vi "V2.4.vi"() -> ()   [LabVIEW 2023]
uses:
  c7928293-0f33-4b54-9085-86d351d5847f.vi
  e7d9e3fd-40eb-4ac7-a8e8-0c749fa94dbf.vi
  <vilib>/Utility/file.llb/Read Delimited Spreadsheet (DBL).vi
  <vilib>/Utility/file.llb/Read Delimited Spreadsheet (string).vi
  <vilib>/Analysis/4window.llb/Symmetric Window (DBL).vi
  <vilib>/Analysis/NI_AAL_SigProc.lvlib
  <vilib>/Analysis/NI_AALPro.lvlib
  <vilib>/Analysis/NI_AALBase.lvlib
panel:
  out "Pics + Index (nvl fct)":dbl[][](array[numeric])
  out "Vallées + Index (nvl fct)":dbl[][](array[numeric])
  out "Var V2V":dbl caption="variance" format="%0.2f"
  out "ET V2V":dbl caption="écart-type" format="%0.2f"
  out "Moy V2V":dbl caption="moyenne" format="%0.2f"
  out "V2V (nvl fct)":dbl[](array[numeric])
  out "Vallées + index DOUBLONS":dbl[][](array[numeric])
  out "var P2P":dbl caption="variance" format="%0.2f"
  out "ET P2P":dbl caption="écart-type" format="%0.2f"
  out "moy P2P":dbl caption="moyenne" format="%0.2f"
  out "P2P (nvl fct) 2":dbl[](array[numeric])
  out "Pics + index DOUBLONS":dbl[][](array[numeric])
  out "Graphe":dbl[](graph)
  out "pente":dbl[](graph)
  out "Pentes":dbl[](array[numeric]) format="%#.6g"
  out "Box moy de 20":dbl[](array[numeric])
  out "Pics Détectés 3":i32 caption="nb trouvé"
  out "Vallées Détectées 3":i32 caption="nb trouvé"
  out "Largeur V":dbl
  out "Seuil V":dbl
  out "Largeur P":dbl
  out "Seuil P":dbl
  out "variance V":dbl caption="variance" format="%0.2f"
  out "standard deviation V":dbl caption="écart-type" format="%0.2f"
  out "mean V":dbl caption="moyenne" format="%0.2f"
  out "Longueur V2V":i32[](array[numeric])
  out "variance P":dbl caption="variance" format="%0.2f"
  out "standard deviation P":dbl caption="écart-type" format="%0.2f"
  out "mean P":dbl caption="moyenne" format="%0.2f"
  out "Longueur P2P":i32[](array[numeric])
  out "Index Vallées":dbl[](array[numeric])
  out "Index Pics":dbl[](array[numeric])
  out "Longueurs SC 2 SC":i32[](graph)
  out "variance":dbl format="%0.2f"
  out "standard deviation 2":dbl caption="écart-type" format="%0.2f"
  out "mean 3":dbl caption="moyenne" format="%0.2f"
  out "First Val of traces":dbl[](array[numeric])
  out "Tableau":dbl[][](array[numeric])
  out "SC1 s":i32[](array[numeric])
  out "Nb de pas (g et dr)":i32
  out "Graphe de signaux mixte":dbl[][](graph)
  out "Cluster":cluster{"SC1":i32, "Aerial":i32, "SC 2":i32}
  out "Longueur de chaque pas (SC 2 SC)":i32[](array[numeric])
  out "Etapes des pas":cluster{"SC1":i32, "Aerial":i32, "SC 2":i32}[](array[cluster])
  out "All data SC/DC/Aerial":string[](array[string])
  out "W condi ?":bool
  out "V target":dbl
  out "Data vitesse et temps":ext[][](array[numeric]) format="%#.5g"
  out "Position graphique Pics/Vallées":cluster{"Locations":dbl[], "Amplitudes":dbl[]}[](graph)
  out "Infos vallées (Fct auto)":cluster{"Locations":dbl[], "Amplitudes":dbl[]}
  out "Infos pics (Fct auto)":cluster{"Locations":dbl[], "Amplitudes":dbl[]}
  # "Val X commence a 20 \ndonc faire -20 pour retrouver data d'une pos"
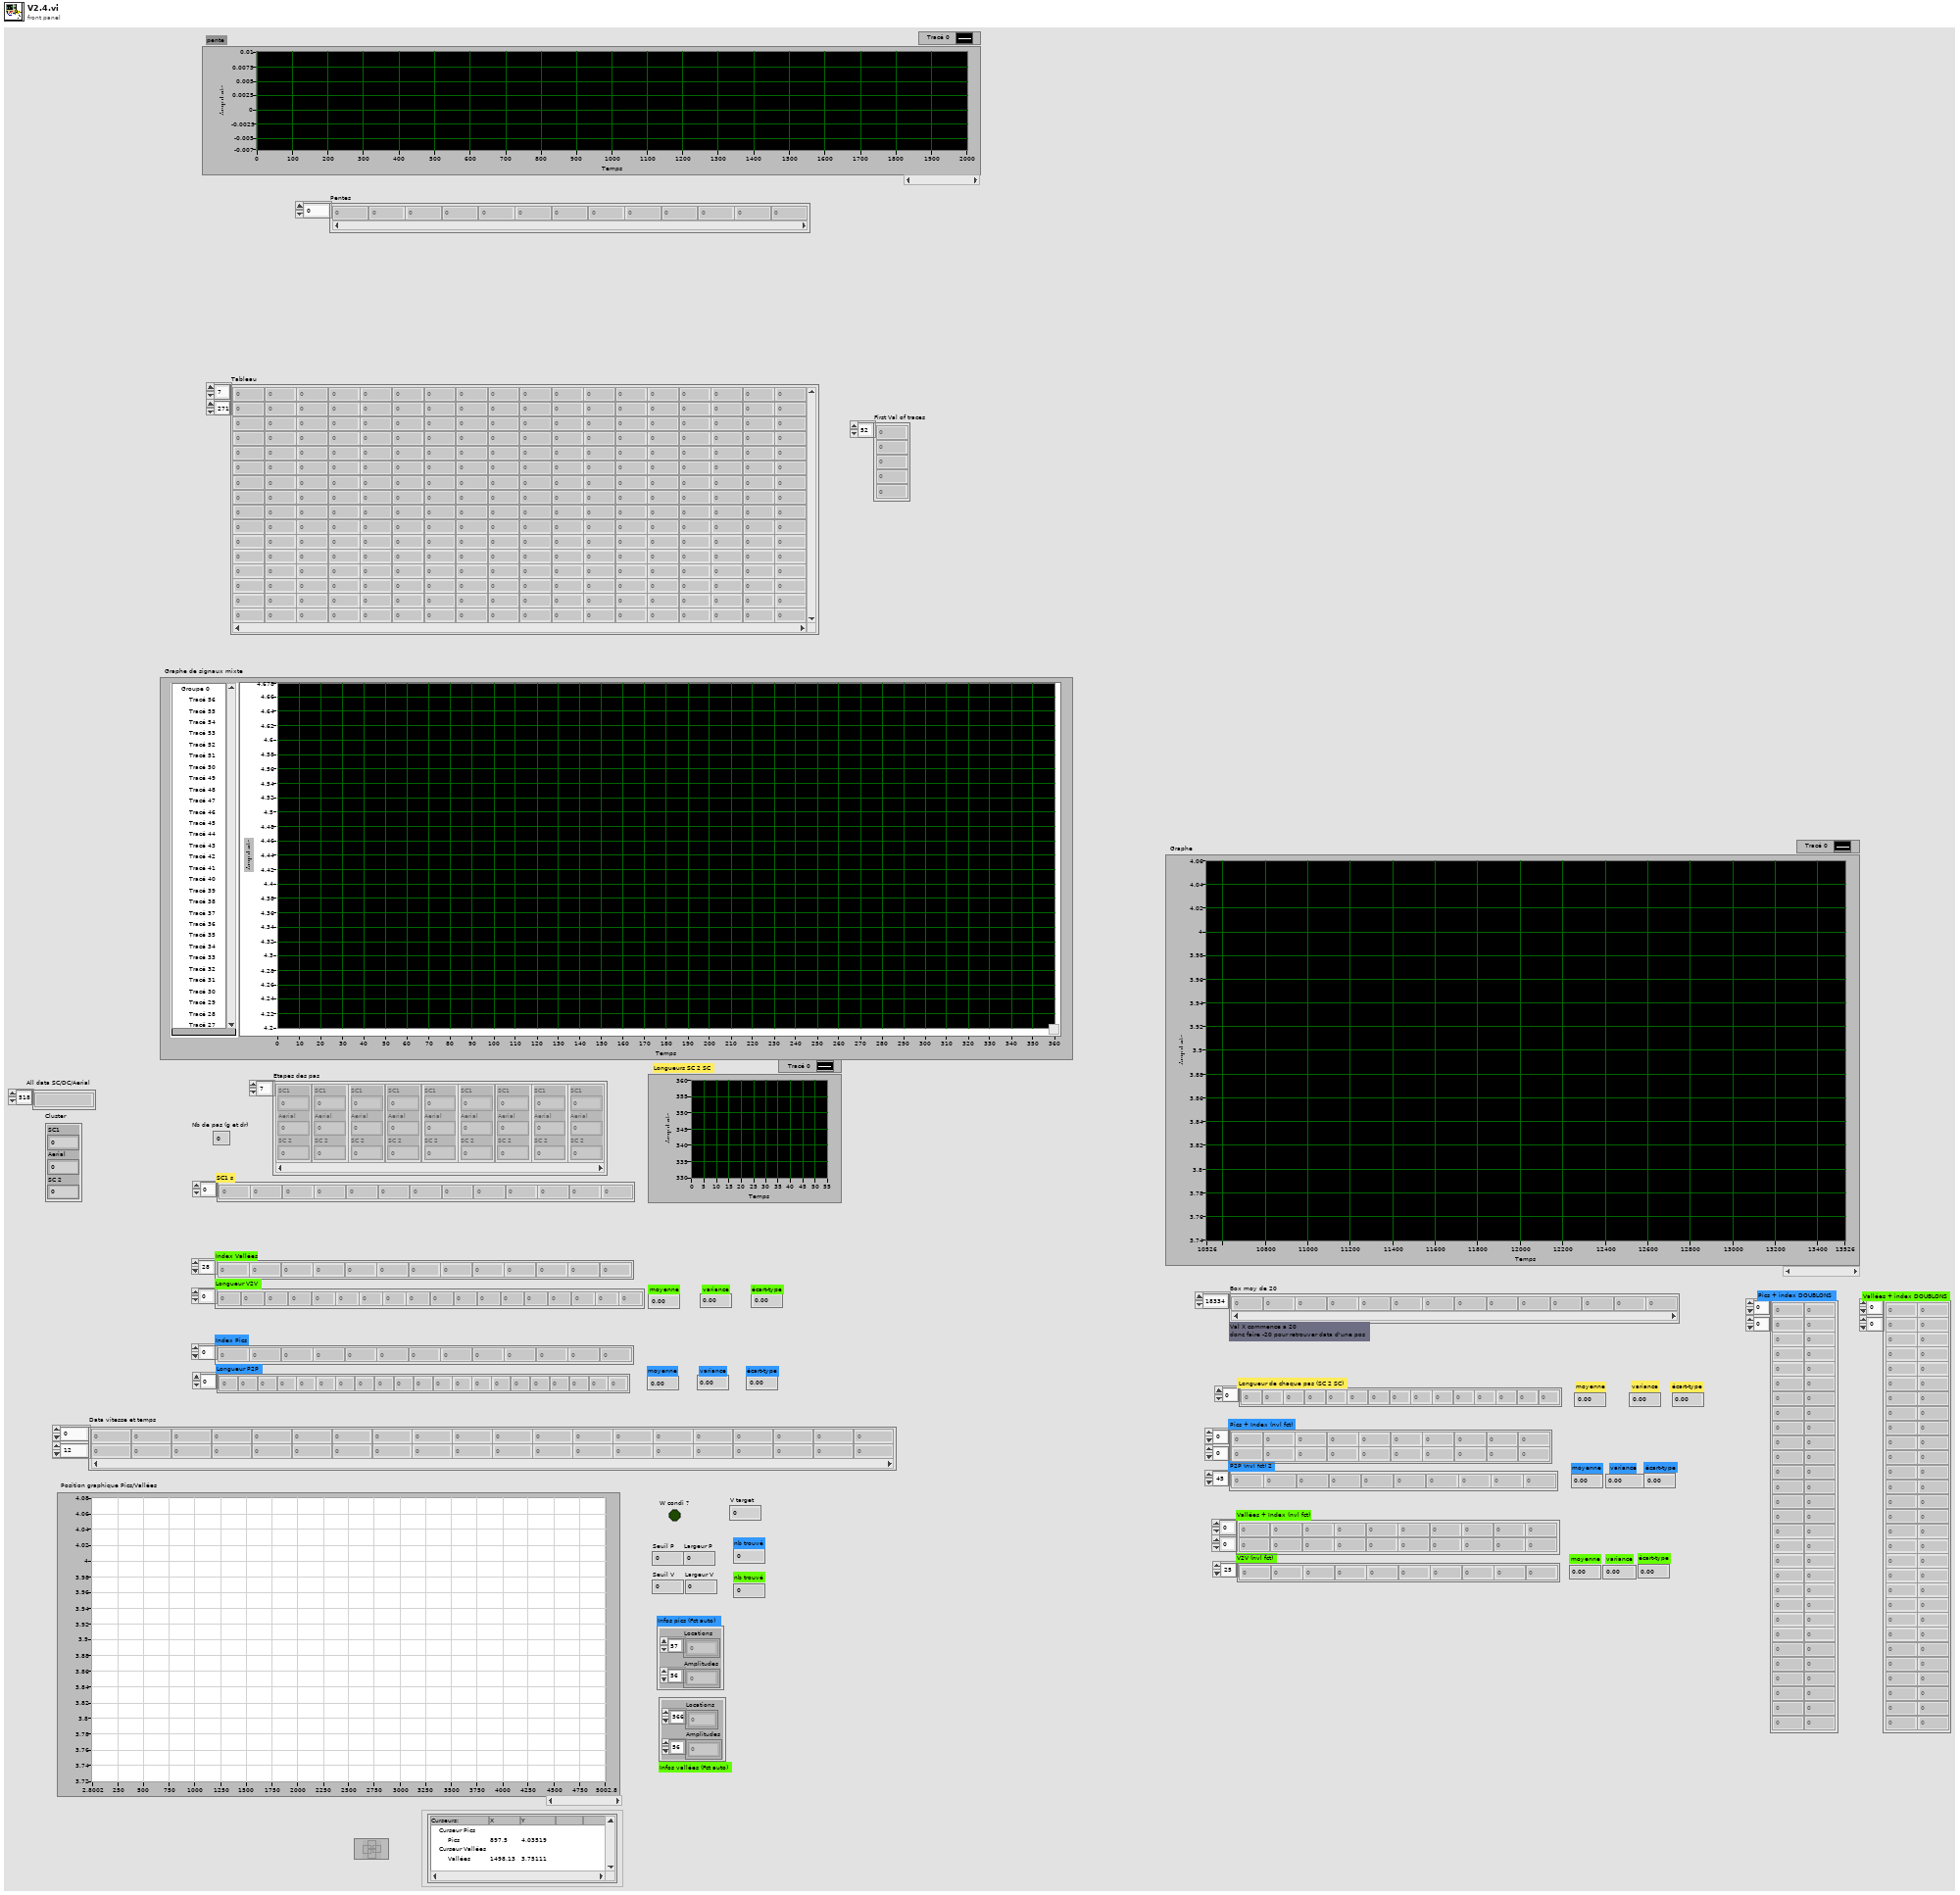
[diagram p1: front panel]
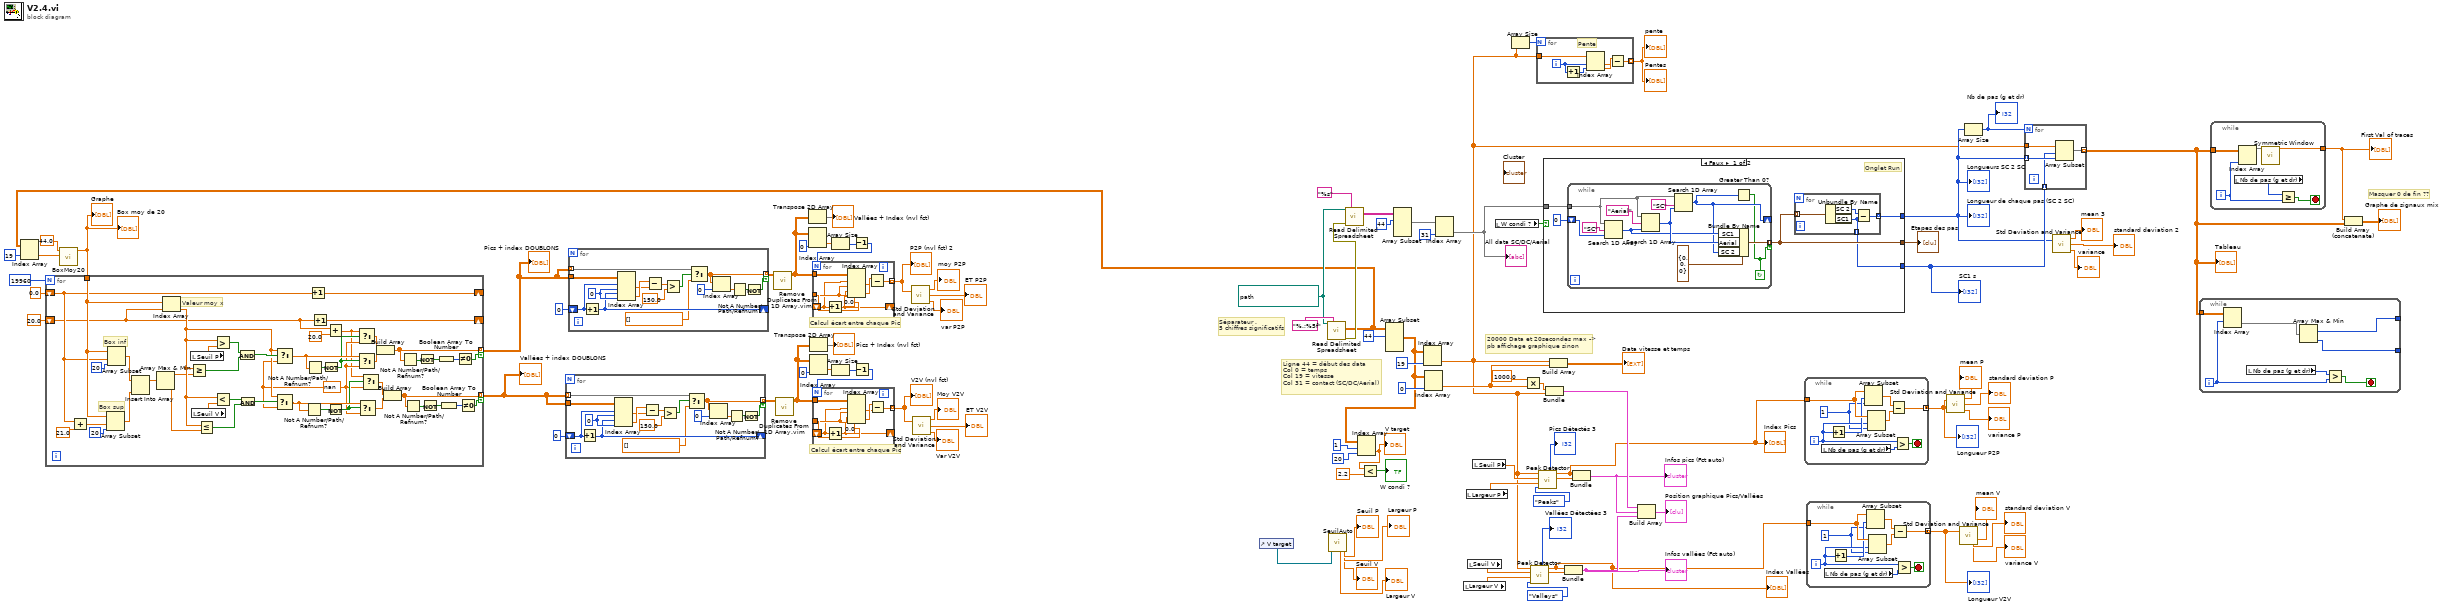
[diagram p0: block diagram]
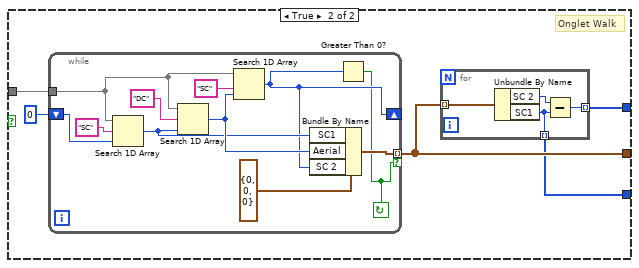
[diagram p2: hidden frame]
diagram:
  w11 = 0.0
  w25 = 0.0
  w77 = path "D:/Documents/Mémoire/Data John Doe/John Doe gaitway 3D locomotion_R14.txt" ("file path (dialog if empty)")
  # "Calcul écart entre chaque Pic"
  # "Calcul écart entre chaque Pic"
  # "Masquer 0 de fin ??"
  # "20000 Data et 20secondes max -> pb affichage graphique sinon"
  # "Séparateur . \n5 chiffres significatifs"
  # "Ligne 44 = début des data\nCol 0 = temps\nCol 19 = vitesse\nCol 31 = contact (SC/DC/Aerial)"
  n1 = control-ref of="V target"() -> (w46:refnum<vi>)
  n2 = call-poly <vilib>:"Read Delimited Spreadsheet.vi"("file path (dialog if empty)"=w77, "format (%.3f)"="%.;%5f") -> ("all rows"=w29:dbl[][], "error out"=w85:errorcluster)  [unwired: 8 in, 4 out]
  n3 = Index Array(array=w29, index (col)=19 ("indice désactivé (col)")) -> (element=w30:dbl[])  [unwired: 1 in]
  n4 = call "BoxMoy20.vi"("all rows"=w30, "Numérique"=44.0) -> ("Tableau 2"=w31:dbl[])  [unwired: 9 in]
  "Box moy de 20" <- w31
  "Graphe" <- w31
  n5 = for {
    N: 19960 -> [_]
    shift-right: [w136] -> _
    shift-left: 0.0 -> [w124]
    tunnel: [w103] -> w15 mode=indexing if=w102
    shift-right: [w133] -> _
    shift-left: 20.0 ("y") -> [w114]
    tunnel: w31 -> [w125]
    tunnel: [w118] -> w27 mode=indexing if=w115
    w105 = nan
    # "Box inf"
    # "Box sup"
    # "Valeur moy x"
    n6 = Add(x=w124, y=21.0) -> (x+y=w140:dbl)
    n7 = Array Subset(array=w125, index=w140, length=20 ("longueur")) -> (w131:dbl[])
    n8 = Array Subset(array=w125, index=w124, length=20 ("longueur")) -> (w132:dbl[])
    n9 = Insert Into Array(array=w132, new element=w131) -> (w130:dbl[])  [unwired: 1 in]
    n10 = Array Max & Min(array=w130) -> (max value=w129:dbl, min value=w128:dbl)  [unwired: 2 out]
    n11 = Index Array(array=w125, index=w114) -> (element=w137:dbl)
    n12 = Greater Or Equal?(x=w137, y=w129) -> (x >= y?=w127:bool)
    n13 = local read "Seuil P"() -> (w139:dbl)
    n14 = local read "Seuil V"() -> (w138:dbl)
    n15 = Less Or Equal?(x=w137, y=w128) -> (x <= y?=w126:bool)
    n16 = Greater?(x=w137, y=w139) -> (0:w145:bool)
    n17 = Less?(x=w137, y=w138) -> (x < y?=w146:bool)
    n18 = And(x=w145, y=w127) -> (x .and. y?=w144:bool)
    n19 = And(x=w146, y=w126) -> (x .and. y?=w147:bool)
    n20 = Select(t=w137, s=w147, f=w105) -> (s? t:f=w107:dbl)
    n21 = Select(t=w137, s=w144, f=w105) -> (s? t:f=w123:dbl)
    n22 = Not A Number/Path/Refnum?(number/path/refnum=w107) -> (NaN/Path/Refnum?=w135:bool)
    n23 = Not A Number/Path/Refnum?(number/path/refnum=w123) -> (NaN/Path/Refnum?=w134:bool)
    n24 = Increment(x=w124) -> (x+1=w136:dbl)
    n25 = Increment(x=w114) -> (x+1=w133:dbl)
    n26 = Not(x=w134) -> (.not. x?=w120:bool)
    n27 = Add(x=w114, y=20.0) -> (x+y=w104:dbl)
    n28 = Not(x=w135) -> (.not. x?=w106:bool)
    n29 = Select(t=w104, s=w120, f=w105) -> (s? t:f=w121:dbl)
    n30 = Select(t=w123, s=w120, f=w105) -> (s? t:f=w122:dbl)
    n31 = Select(t=w107, s=w106, f=w105) -> (s? t:f=w112:dbl)
    n32 = Select(t=w104, s=w106, f=w105) -> (s? t:f=w111:dbl)
    n33 = Build Array(w121, w122) -> (w118:dbl[])
    n34 = Build Array(w111, w112) -> (w103:dbl[])
    n35 = Not A Number/Path/Refnum?(number/path/refnum=w118) -> (NaN/Path/Refnum?=w119:bool[])
    n36 = Not A Number/Path/Refnum?(number/path/refnum=w103) -> (NaN/Path/Refnum?=w110:bool[])
    n37 = Not(x=w119) -> (.not. x?=w117:bool[])
    n38 = Not(x=w110) -> (.not. x?=w109:bool[])
    n39 = Boolean Array To Number(Boolean array=w117) -> (number=w116:u32)
    n40 = Boolean Array To Number(Boolean array=w109) -> (number=w108:u32)
    n41 = Not Equal To 0?(x=w116) -> (x != 0?=w115:bool)
    n42 = Not Equal To 0?(x=w108) -> (x != 0?=w102:bool)
  }
  "Pics + index DOUBLONS" <- w27
  "Vallées + index DOUBLONS" <- w15
  n43 = for {
    tunnel: w15 -> [w163]
    shift-right: [w160] -> _
    shift-left: 0 -> [w161]
    tunnel: w15 -> [w156] mode=indexing
    tunnel: [w153] -> w6 mode=indexing if=w151
    w162 = 0 ("indice (col)")
    n44 = Increment(x=w161) -> (x+1=w160:i32)
    n45 = Index Array(array=w163, index (row) #1=w161, index (col) #1=w162, index (row) #2=w160, index (col) #2=w162) -> (element #1=w149:dbl, element #2=w150:dbl)
    n46 = Subtract(x=w150, y=w149) -> (x-y=w159:dbl)
    n47 = Greater?(x=w159, y=150.0) -> (0:w157:bool)
    n48 = Select(t=w156, s=w157, f=dbl[] []) -> (s? t:f=w153:dbl[])
    n49 = Index Array(array=w153, index=0 ("indice")) -> (element=w152:dbl)
    n50 = Not A Number/Path/Refnum?(number/path/refnum=w152) -> (NaN/Path/Refnum?=w154:bool)
    n51 = Not(x=w154) -> (.not. x?=w151:bool)
  }
  n52 = for {
    tunnel: w27 -> [w179]
    shift-right: [w176] -> _
    shift-left: 0 -> [w177]
    tunnel: w27 -> [w172] mode=indexing
    tunnel: [w169] -> w26 mode=indexing if=w167
    w178 = 0 ("indice (col)")
    n53 = Increment(x=w177) -> (x+1=w176:i32)
    n54 = Index Array(array=w179, index (row) #1=w177, index (col) #1=w178, index (row) #2=w176, index (col) #2=w178) -> (element #1=w165:dbl, element #2=w166:dbl)
    n55 = Subtract(x=w166, y=w165) -> (x-y=w175:dbl)
    n56 = Greater?(x=w175, y=150.0) -> (0:w173:bool)
    n57 = Select(t=w172, s=w173, f=dbl[] []) -> (s? t:f=w169:dbl[])
    n58 = Index Array(array=w169, index=0 ("indice")) -> (element=w168:dbl)
    n59 = Not A Number/Path/Refnum?(number/path/refnum=w168) -> (NaN/Path/Refnum?=w170:bool)
    n60 = Not(x=w170) -> (.not. x?=w167:bool)
  }
  n61 = call "Remove Duplicates From 1D Array.vim"("array"=w26) -> ("array with duplicates removed"=w4:dbl[][])  [unwired: 10 in]
  n62 = call "Remove Duplicates From 1D Array.vim"("array"=w6) -> ("array with duplicates removed"=w2:dbl[][])  [unwired: 10 in]
  n63 = Transpose 2D Array(2D array=w4) -> (transposed array=→"Vallées + Index (nvl fct)":dbl[][])
  n64 = Index Array(array=w4, index (col)=0 ("indice (col)")) -> (element=w19:dbl[])  [unwired: 1 in]
  n65 = Transpose 2D Array(2D array=w2) -> (transposed array=→"Pics + Index (nvl fct)":dbl[][])
  n66 = Index Array(array=w2, index (col)=0 ("indice (col)")) -> (element=w9:dbl[])  [unwired: 1 in]
  n67 = Array Size(array=w19) -> (size(s)=w18:i32)
  n68 = Array Size(array=w9) -> (size(s)=w8:i32)
  n69 = Decrement(x=w18) -> (x-1=w17:i32)
  n70 = for {
    N: w17 -> [_]
    tunnel: w4 -> [w184]
    shift-right: [w180] -> _
    shift-left: w25 -> [w181]
    tunnel: w25 -> [w182]
    tunnel: [w183] -> w24 mode=indexing
    n71 = Increment(x=w181) -> (x+1=w180:dbl)
    n72 = Index Array(array=w184, index (row) #1=w181, index (col) #1=w182, index (row) #2=w180, index (col) #2=w182) -> (element #1=w185:dbl, element #2=w186:dbl)
    n73 = Subtract(x=w186, y=w185) -> (x-y=w183:dbl)
  }
  "P2P (nvl fct) 2" <- w24
  n74 = Decrement(x=w8) -> (x-1=w7:i32)
  n75 = for {
    N: w7 -> [_]
    tunnel: w2 -> [w191]
    shift-right: [w187] -> _
    shift-left: w11 -> [w188]
    tunnel: w11 -> [w189]
    tunnel: [w190] -> w5 mode=indexing
    n76 = Increment(x=w188) -> (x+1=w187:dbl)
    n77 = Index Array(array=w191, index (row) #1=w188, index (col) #1=w189, index (row) #2=w187, index (col) #2=w189) -> (element #1=w192:dbl, element #2=w193:dbl)
    n78 = Subtract(x=w193, y=w192) -> (x-y=w190:dbl)
  }
  "V2V (nvl fct)" <- w5
  n79 = call <vilib>:"Std Deviation and Variance.vi"("X"=w24) -> ("mean"=→"moy P2P":dbl, "standard deviation"=→"ET P2P":dbl, "variance"=→"var P2P":dbl)  [unwired: 1 in]
  n80 = call <vilib>:"Std Deviation and Variance.vi"("X"=w5) -> ("mean"=→"Moy V2V":dbl, "standard deviation"=→"ET V2V":dbl, "variance"=→"Var V2V":dbl)  [unwired: 1 in]
  n81 = call "SeuilAuto.vi"("V target"=w46) -> ("Seuil V"=→"Seuil V":dbl, "Largeur P"=→"Largeur P":dbl, "Seuil P"=→"Seuil P":dbl, "Largeur V"=→"Largeur V":dbl)  [unwired: 7 in]
  n82 = call-poly <vilib>:"Read Delimited Spreadsheet.vi"("file path (dialog if empty)"=w77, "format (%s)"="%s" ("format (%.3f)"), "error in (no error)"=w85) -> ("all rows"=w84:string[][])  [unwired: 7 in, 5 out]
  n83 = Array Subset(array=w29, index (row)=44 ("indice")) -> (w87:dbl[][])  [unwired: 3 in]
  n84 = Index Array(array=w87, index (row)=1 ("indice (ligne)"), index (col)=20 ("indice (col)")) -> (element=w92:dbl)
  "V target" <- w92
  n85 = Less?(x=w92, y=2.2) -> (x < y?=→"W condi ?":bool)
  n86 = Array Subset(array=w84, index (row)=44 ("indice")) -> (w83:string[][])  [unwired: 3 in]
  n87 = Index Array(array=w87, index (col)=19 ("indice (col)")) -> (element=w34:dbl[])  [unwired: 1 in]
  n88 = Index Array(array=w87, index (col)=0 ("indice (col)")) -> (element=w88:dbl[])  [unwired: 1 in]
  n89 = Index Array(array=w83, index (col)=31 ("indice (col)")) -> (element=w80:string[])  [unwired: 1 in]
  "All data SC/DC/Aerial" <- w80
  n90 = local read "Largeur V"() -> (w55:dbl)
  n91 = local read "Largeur P"() -> (w53:dbl)
  n92 = local read "Seuil V"() -> (w56:dbl)
  n93 = local read "Seuil P"() -> (w54:dbl)
  n94 = local read "W condi ?"() -> (w69:bool)
  n95 = Array Size(array=w34) -> (size(s)=w35:i32)
  n96 = Multiply(x=1000.0, y=w88) -> (x*y=w89:dbl[])
  n97 = call <vilib>:"Peak Detector.vi"("peaks/valleys"=enum32{"Peaks", "Valleys"}."Valleys", "width"=w55, "threshold"=w56, "X"=w34) -> ("Amplitudes"=w60:dbl[], "Locations"=w49:dbl[], "# found"=→"Vallées Détectées 3":i32)  [unwired: 3 in, 2 out]
  "Index Vallées" <- w49
  n98 = for {
    N: w35 -> [_]
    tunnel: w34 -> [w199]
    tunnel: [w195] -> w33 mode=indexing
    i -> [w194]
    # "Pente"
    n99 = Increment(x=w194) -> (x+1=w198:i32)
    n100 = Index Array(array=w199, index #1=w194, index #2=w198) -> (element #1=w196:dbl, element #2=w197:dbl)
    n101 = Subtract(x=w197, y=w196) -> (x-y=w195:dbl)
  }
  "Pentes" <- w33
  "pente" <- w33
  n102 = call <vilib>:"Peak Detector.vi"("peaks/valleys"=enum32{"Peaks", "Valleys"}."Peaks", "width"=w53, "threshold"=w54, "X"=w34) -> ("Amplitudes"=w58:dbl[], "Locations"=w51:dbl[], "# found"=→"Pics Détectés 3":i32)  [unwired: 3 in, 2 out]
  "Index Pics" <- w51
  n103 = case shown="Faux" w69 {
    tunnel: w80 -> [w203 w224]
    tunnel: [w201 w222] -> w78
    tunnel: [w202 w221] -> w70
    tunnel: [w200 w220] -> w76
    frame False {
      # "Onglet Run"
      n104 = while {
        tunnel: [w217] -> w201 mode=indexing if=w209
        tunnel: w203 -> [w213]
        shift-right: [w210] -> _
        shift-left: 0 -> [w212]
        stop <- w209 continue-if-true
        n105 = Search 1D Array(1D array=w213, element="SC" ("élément"), start index (0)=w212) -> (index of element=w211:i32)
        n106 = Search 1D Array(1D array=w213, element="Aerial" ("élément"), start index (0)=w211) -> (index of element=w219:i32)
        n107 = Search 1D Array(1D array=w213, element="SC" ("élément"), start index (0)=w219) -> (index of element=w210:i32)
        n108 = Bundle By Name(cluster=cluster{"SC1":i32, "Aerial":i32, "SC 2":i32} {"SC1"=0, "Aerial"=0, "SC 2"=0} ("Cluster"), "SC1"=w211, "Aerial"=w219, "SC 2"=w210) -> (w217:cluster{"SC1":i32, "Aerial":i32, "SC 2":i32})
        n109 = Greater Than 0?(x=w210) -> (x > 0?=w209:bool)
      }
      n110 = for {
        tunnel: w201 -> [w208] mode=indexing
        tunnel: [w206] -> w202 mode=indexing
        tunnel: [w205] -> w200 mode=indexing
        n111 = Unbundle By Name(w208) -> ("SC 2"=w207:i32, "SC1"=w205:i32)
        n112 = Subtract(x=w207, y=w205) -> (x-y=w206:i32)
      }
    }
    frame True {
      # "Onglet Walk"
      n113 = while {
        tunnel: [w237] -> w222 mode=indexing if=w229
        tunnel: w224 -> [w233]
        shift-right: [w230] -> _
        shift-left: 0 -> [w232]
        stop <- w229 continue-if-true
        n114 = Search 1D Array(1D array=w233, element="SC" ("élément"), start index (0)=w232) -> (index of element=w231:i32)
        n115 = Search 1D Array(1D array=w233, element="DC" ("élément"), start index (0)=w231) -> (index of element=w239:i32)
        n116 = Search 1D Array(1D array=w233, element="SC" ("élément"), start index (0)=w239) -> (index of element=w230:i32)
        n117 = Bundle By Name(cluster=cluster{"SC1":i32, "Aerial":i32, "SC 2":i32} {"SC1"=0, "Aerial"=0, "SC 2"=0} ("Cluster"), "SC1"=w231, "Aerial"=w239, "SC 2"=w230) -> (w237:cluster{"SC1":i32, "Aerial":i32, "SC 2":i32})
        n118 = Greater Than 0?(x=w230) -> (x > 0?=w229:bool)
      }
      n119 = for {
        tunnel: w222 -> [w228] mode=indexing
        tunnel: [w226] -> w221 mode=indexing
        tunnel: [w225] -> w220 mode=indexing
        n120 = Unbundle By Name(w228) -> ("SC 2"=w227:i32, "SC1"=w225:i32)
        n121 = Subtract(x=w227, y=w225) -> (x-y=w226:i32)
      }
    }
  }
  "Etapes des pas" <- w78
  "Longueur de chaque pas (SC 2 SC)" <- w70
  "SC1 s" <- w76
  "Longueurs SC 2 SC" <- w70
  n122 = Bundle(w89, w34) -> (w97:cluster{dbl[], dbl[]})  [unwired: 1 in]
  n123 = Build Array(w34, w88) -> (→"Data vitesse et temps":dbl[][])
  n124 = Bundle("Locations"=w49, "Amplitudes"=w60) -> (w50:cluster{"Locations":dbl[], "Amplitudes":dbl[]})  [unwired: 1 in]
  "Infos vallées (Fct auto)" <- w50
  n125 = Bundle("Locations"=w51, "Amplitudes"=w58) -> (w52:cluster{"Locations":dbl[], "Amplitudes":dbl[]})  [unwired: 1 in]
  "Infos pics (Fct auto)" <- w52
  n126 = Build Array(w97, w52, w50) -> (→"Position graphique Pics/Vallées":cluster{"Locations":dbl[], "Amplitudes":dbl[]}[])
  n127 = while {
    tunnel: w51 -> [w245]
    tunnel: [w248] -> w68 mode=concatenating
    i -> [w243]
    stop <- w247 stop-if-true
    w242 = 1 ("longueur")
    n128 = local read "Nb de pas (g et dr)"() -> (w246:i32)
    n129 = Increment(x=w243) -> (x+1=w244:i32)
    n130 = Array Subset(array=w245, index=w244, length=w242) -> (w241:dbl[])
    n131 = Array Subset(array=w245, index=w243, length=w242) -> (w240:dbl[])
    n132 = Subtract(x=w241, y=w240) -> (x-y=w248:dbl[])
    n133 = Greater?(x=w243, y=w246) -> (0:w247:bool)
  }
  "Longueur P2P" <- w68
  n134 = while {
    tunnel: w49 -> [w255]
    tunnel: [w257] -> w64 mode=concatenating
    i -> [w253]
    stop <- w256 stop-if-true
    w252 = 1 ("longueur")
    n135 = local read "Nb de pas (g et dr)"() -> (w249:i32)
    n136 = Increment(x=w253) -> (x+1=w254:i32)
    n137 = Array Subset(array=w255, index=w254, length=w252) -> (w251:dbl[])
    n138 = Array Subset(array=w255, index=w253, length=w252) -> (w250:dbl[])
    n139 = Subtract(x=w251, y=w250) -> (x-y=w257:dbl[])
    n140 = Greater?(x=w253, y=w249) -> (0:w256:bool)
  }
  "Longueur V2V" <- w64
  n141 = call <vilib>:"Std Deviation and Variance.vi"("X"=w68) -> ("mean"=→"mean P":dbl, "standard deviation"=→"standard deviation P":dbl, "variance"=→"variance P":dbl)  [unwired: 1 in]
  n142 = call <vilib>:"Std Deviation and Variance.vi"("X"=w64) -> ("mean"=→"mean V":dbl, "standard deviation"=→"standard deviation V":dbl, "variance"=→"variance V":dbl)  [unwired: 1 in]
  n143 = Array Size(array=w70) -> (size(s)=w75:i32)
  "Nb de pas (g et dr)" <- w75
  n144 = for {
    N: w75 -> [_]
    tunnel: w34 -> [w259]
    tunnel: w70 -> [w261] mode=indexing
    tunnel: w76 -> [w260] mode=indexing
    tunnel: [w258] -> w37 mode=indexing
    n145 = Array Subset(array=w259, index=w260, length=w261) -> (w258:dbl[])
  }
  "Tableau" <- w37
  n146 = call <vilib>:"Std Deviation and Variance.vi"("X"=w70) -> ("mean"=→"mean 3":dbl, "standard deviation"=→"standard deviation 2":dbl, "variance"=→"variance":dbl)  [unwired: 1 in]
  n147 = while {
    tunnel: w37 -> [w268]
    tunnel: [w263] -> _
    tunnel: [w262] -> _
    i -> [w267]
    stop <- w265 stop-if-true
    n148 = Index Array(array=w268, index (row)=w267) -> (element=w264:dbl[])  [unwired: 1 in]
    n149 = local read "Nb de pas (g et dr)"() -> (w266:i32)
    n150 = Array Max & Min(array=w264) -> (max index (indices)=w263:i32, min index (indices)=w262:i32)  [unwired: 2 out]
    n151 = Greater?(x=w266, y=w267) -> (0:w265:bool)
  }
  n152 = while {
    tunnel: w37 -> [w274]
    tunnel: [w272] -> w74
    i -> [w270]
    stop <- w269 stop-if-true
    n153 = local read "Nb de pas (g et dr)"() -> (w271:i32)
    n154 = Index Array(array=w274, index (col)=w270) -> (element=w273:dbl[])  [unwired: 1 in]
    n155 = call-poly <vilib>:"Symmetric Window.vi"("X"=w273) -> ("Windowed X"=w272:dbl[])  [unwired: 9 in, 1 out]
    n156 = Greater Or Equal?(x=w271, y=w270) -> (x >= y?=w269:bool)
  }
  "First Val of traces" <- w74
  n157 = Build Array (concatenate)(w74, w37) -> (→"Graphe de signaux mixte":dbl[][])
